vi "GetWireReference.vi"(6 "error in":errorcluster, 9 "wire in":refnum<class "Wire.lvclass">) -> (0 "error out":errorcluster, 1 "reference out":refnum<vi>, 3 "wire out":refnum<class "Wire.lvclass">)   [LabVIEW 2014, in "Raspberry Pi Compatible Compiler for LabVIEW.lvlib" / "Wire.lvclass"]
uses:
  Wire.lvclass
  Generic/Generic.lvclass
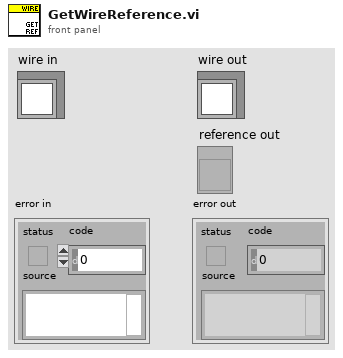
[diagram p1: front panel]
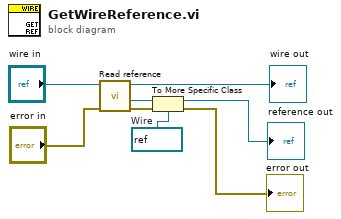
[diagram p0: block diagram]
diagram:
  w4 = refnum<vi> refnum  # Wire
  n1 = call "Read reference.vi"("error in"="error in", "GObject in"="wire in") -> ("error out"=w5:errorcluster, "reference"=w6:refnum<vi>, "GObject out"=→"wire out":refnum<class "Wire.lvclass">)  [unwired: 5 in]
  n2 = To More Specific Class(target class=w4, reference=w6, error in=w5) -> (specific class reference=→"reference out":refnum<vi>, error out=→"error out":errorcluster)
